vi "View AP Data.vi"() -> ()   [LabVIEW 2018]
panel:
  out "Waveform Graph 6":i16[][](graph)
  out "name":string
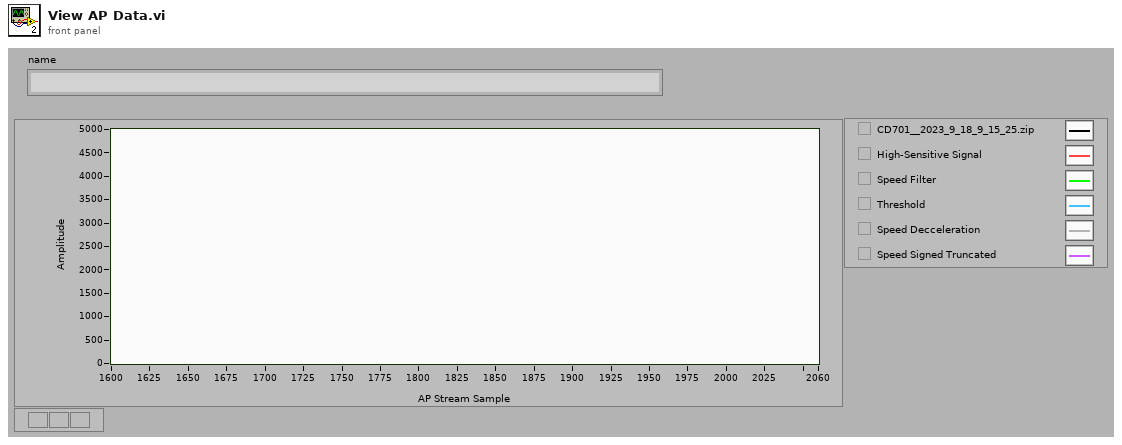
[diagram p1: front panel]
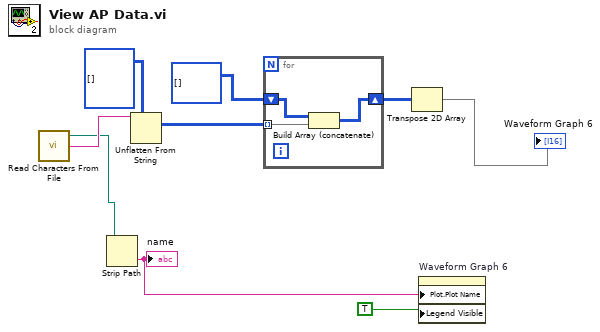
[diagram p0: block diagram]
diagram:
  n1 = call <vilib>:"Read Characters From File.vi"() -> ("new file path (NotAPath if cancelled)"=w2:path, "character string"=w9:string)  [unwired: 6 in, 2 out]
  n2 = Strip Path(path=w2) -> (name=w1:string)  [unwired: 1 out]
  "name" <- w1
  n3 = Unflatten From String(type=i16[][][] [] ("AP Data"), binary string=w9) -> (value=w7:i16[][][])  [unwired: 3 in, 2 out]
  n4 = for {
    tunnel: w7 -> [w10] mode=indexing
    shift-right: [w12] -> w5
    shift-left: i16[][] [] -> [w11]
    n5 = Build Array (concatenate)(w11, w10) -> (w12:i16[][])
  }
  n6 = Transpose 2D Array(2D array=w5) -> (transposed array=→"Waveform Graph 6":i16[][])
  n7 = property on="Waveform Graph 6" class="WFGraph (严格)"("Plot.Plot Name"=w1, "Legend Visible"=TRUE ("Legend:Visible")) -> ()  [unwired: 2 in, 2 out]
